vi "User_event.vi"() -> ()   [LabVIEW 2019]
panel:
  out "userevent":refnum<user-event>
  out "Error Out":errorcluster
  in  "Error In":errorcluster
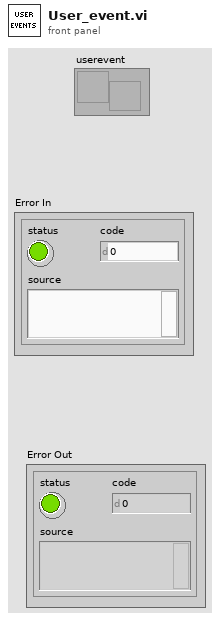
[diagram p1: front panel]
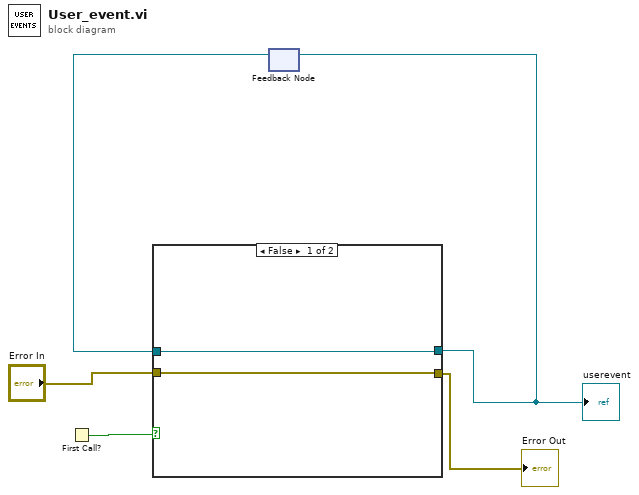
[diagram p0: block diagram]
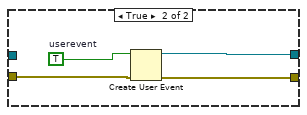
[diagram p2: hidden frame]
diagram:
  n1 = First Call?() -> (First Call?: T/F=w5:bool)
  n2 = feedback #1() -> (w4:refnum<user-event>)  [unwired: 1 in]
  n3 = case shown="False" w5 {
    tunnel: [w7 w10] -> w3
    tunnel: w4 -> [w7 _]
    tunnel: "Error In" -> [w6 w9]
    tunnel: [w6 w8] -> w1
    frame False {
    }
    frame True {
      w11 = TRUE  # userevent
      n4 = Create User Event(user event datatype=w11, error in=w9) -> (user event=w10:refnum<user-event>, error out=w8:errorcluster)
    }
  }
  "userevent" <- w3
  "Error Out" <- w1
  n5 = feedback-in #1(w3) -> ()
